vi "Mutate_v1_to_v2.vi"(11 "SerializableData_v1":T2) -> (0 "error out":errorcluster, 3 "SerializableData_v2":T1)   [LabVIEW 2019, in "Hulk Hogan.lvclass"]
uses:
  Hulk Hogan.lvclass
  SerializableData_v1.ctl
  SerializableData_v2.ctl
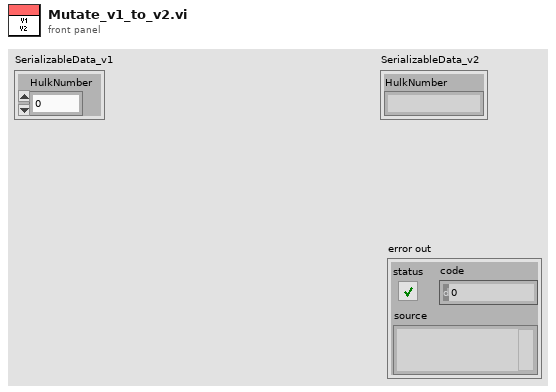
[diagram p1: front panel]
types:
  T1 = typedef "Hulk Hogan.lvclass/SerializableData_v2.ctl" = cluster{"HulkNumber":string}
  T2 = typedef "Hulk Hogan.lvclass/SerializableData_v1.ctl" = cluster{"HulkNumber":dbl}
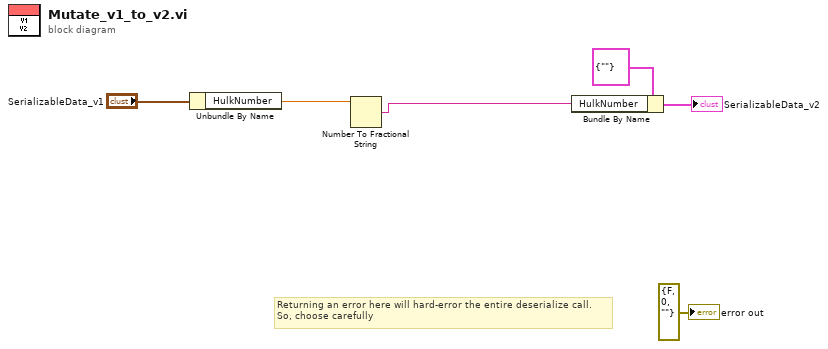
[diagram p0: block diagram]
diagram:
  # "Returning an error here will hard-error the entire deserialize call.\nSo, choose carefully"
  n1 = Unbundle By Name("SerializableData_v1") -> ("HulkNumber"=w3:dbl)
  n2 = Number To Fractional String(number=w3) -> (F-format string=w2:string)  [unwired: 3 in]
  n3 = Bundle By Name(cluster=T1 {"HulkNumber"=""} ("SerializableData"), "HulkNumber"=w2) -> (→"SerializableData_v2":T1)
  "error out" <- errorcluster {"status"=FALSE, "code"=0, "source"=""} ("error out")
